vi "TestDownlink.vi"(1 "DL Tx  Power":dbl=-100.0, 2 "FPGA Reference":refnum<k20>, 3 "DL Data Rate":dbl=600.0 format="%.2f", 4 "DL Tx Freq":i64=905193250, 5 "error in":errorcluster {"code" format="%.0x"}, 6 "DL Rx Timeout (ms)":u32=60, 7 "Resp Timeout (ms)":i32 min=0, 9 "SMU Reference in":refnum<k15>, 10 "DL Rx Freq (Hz)":i64=905200000, 11 "Active Dut":T1, 12 "DL Freq Offset (Hz)":i64=6750, 13 "DxSupply":string="0") -> (14 "Set DL OK":bool, 15 "DL RSSI (dBm)":i16, 16 "Received Text":string, 17 "Get DL OK":bool, 18 "Meas DL Idd":dbl format="%0.5f", 19 "error out":errorcluster)   [LabVIEW 2018]
uses:
  Resources_Test/UART/ControlTestSlot.ctl
  <instrlib>/niRFSG/niRFSG.llb/niRFSG Ref Clock Sources.ctl
panel:
  out "Loop Index":i32
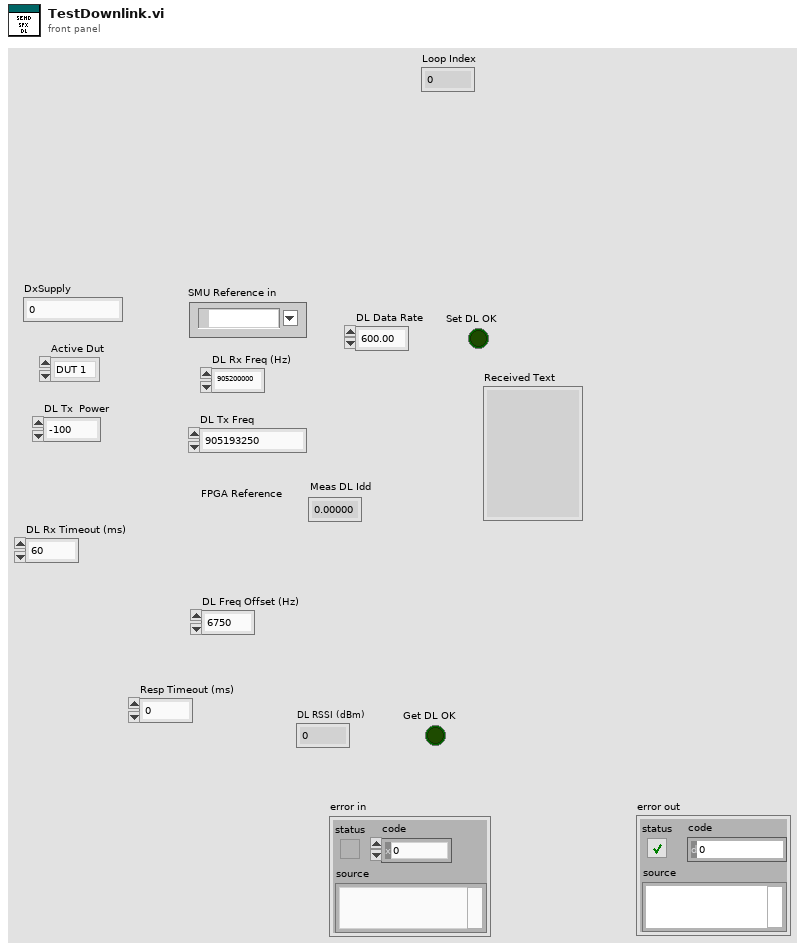
[diagram p1: front panel]
types:
  T1 = typedef "ControlTestSlot.ctl" = enum16{"DUT 1", "DUT 2"}
  T2 = typedef "niRFSG Ref Clock Sources.ctl" = string
  T3 = typedef "niAMT.lvlib/Complex Data Waveform.ctl" = cluster{"t0":dbl, "dt":dbl, "Y":cdb[]}
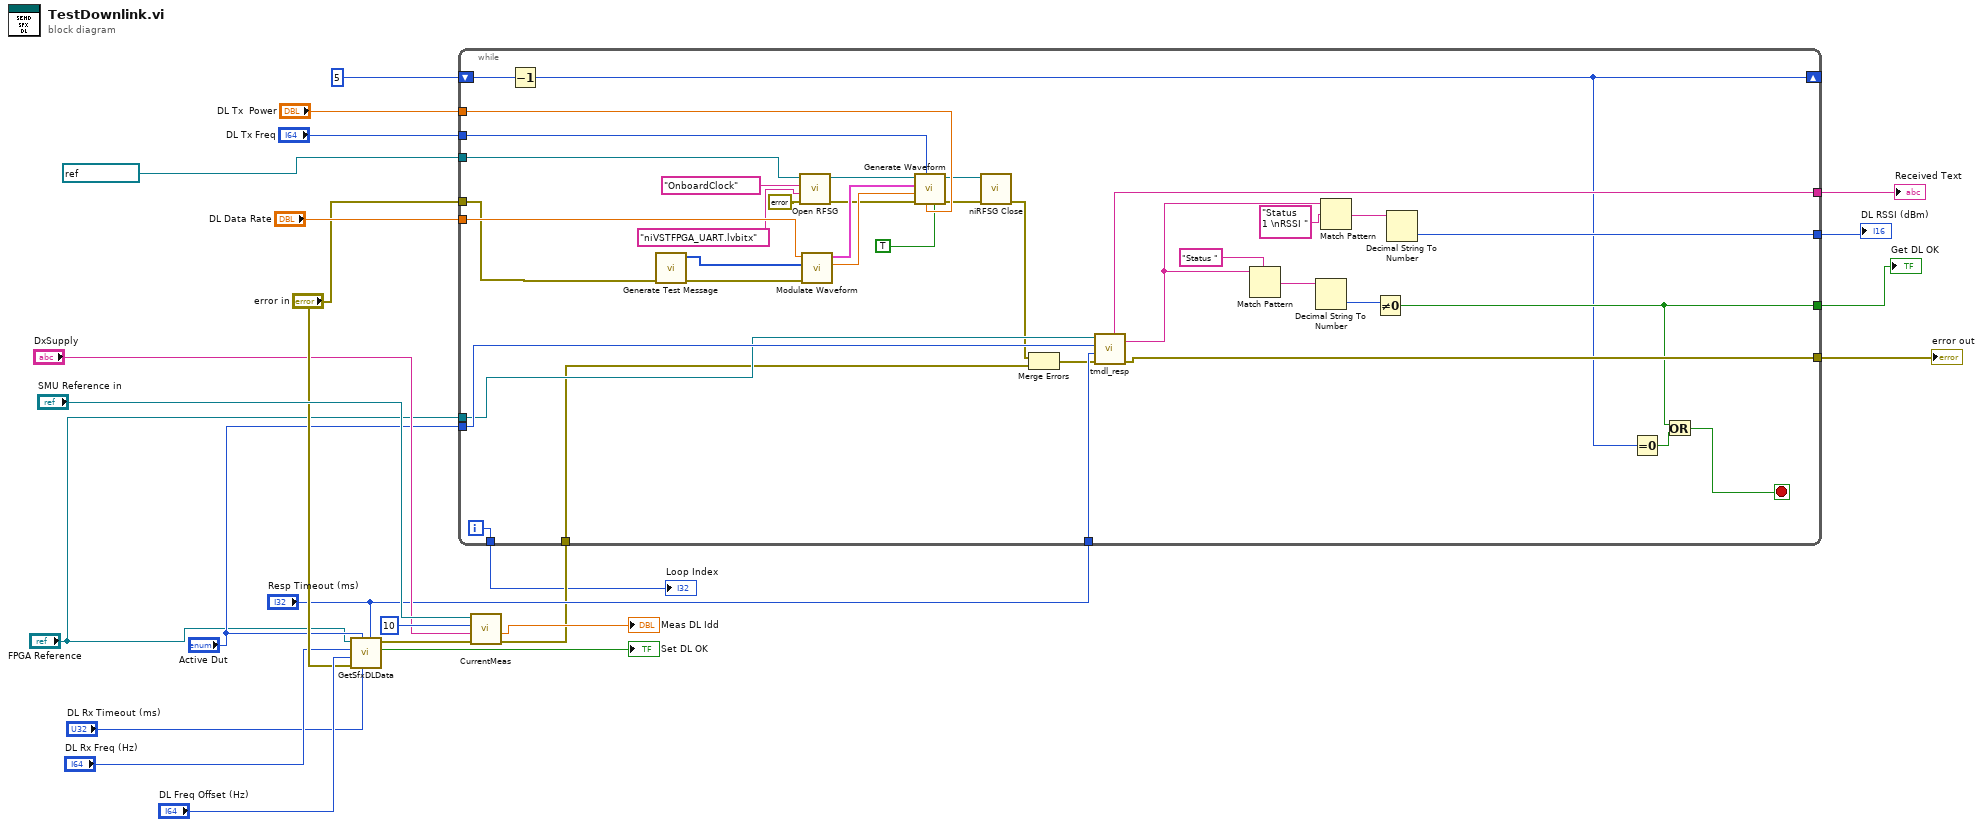
[diagram p0: block diagram]
diagram:
  n1 = call "GetSfxDLData.vi"("Resp Timeout (ms)"="Resp Timeout (ms)", "Rx Timeout (ms)"="DL Rx Timeout (ms)", "Enum"="Active Dut", "Error In"="error in", "Freq Offset (Hz)"="DL Freq Offset (Hz)", "Rx Freq (Hz)"="DL Rx Freq (Hz)", "FPGA Reference"="FPGA Reference") -> ("Error Out"=w20:errorcluster, "Get DL OK"=→"Set DL OK":bool)  [unwired: 3 out]
  n2 = call "CurrentMeas.vi"("error in (no error)"=w20, "DxSupply"="DxSupply", "Measure Record Length"=10, "instrument handle"="SMU Reference in") -> ("error out"=w7:errorcluster, "Idd Peak"=→"Meas DL Idd":dbl)  [unwired: 4 in, 2 out]
  n3 = while {
    tunnel: "DL Tx  Power" -> [w61]
    tunnel: "DL Data Rate" -> [w60]
    tunnel: "DL Tx Freq" -> [w59]
    tunnel: refnum<k15> "PXI1Slot5" ("RFSG Reference in") -> [w58]
    tunnel: "error in" -> [w57]
    tunnel: "Resp Timeout (ms)" -> [w55]
    tunnel: "Active Dut" -> [w54]
    tunnel: "FPGA Reference" -> [w53]
    tunnel: w7 -> [w52]
    tunnel: [w30] -> w5
    tunnel: [w29] -> w4
    tunnel: [w28] -> w3
    tunnel: [w27] -> w2
    shift-right: [w26] -> _
    shift-left: 5 -> [w32]
    tunnel: [w25] -> w1
    i -> [w25]
    stop <- w56 stop-if-true
    n4 = Decrement(x=w32) -> (x-1=w26:i32)
    n5 = call "Generate Test Message.vi"("error in"=w57) -> ("error out"=w41:errorcluster, "Output Bit Stream"=w40:i8[])  [unwired: 9 in]
    n6 = call "Open RFSG.vi"("error in"=errorcluster {"status"=FALSE, "code"=0, "source"=""}, "Bitfile"="niVSTFPGA_UART.lvbitx" ("Option String"), "Clock Source"=T2 "OnboardClock", "Resource Name"=w58) -> ("error out"=w47:errorcluster, "IVI Refnum out"=w46:refnum<k15>)  [unwired: 6 in]
    n7 = call "Modulate Waveform.vi"("error in"=w41, "input bit stream"=w40, "Symbol Rate, Hz"=w60) -> ("Signal Bandwidth"=w51:dbl, "output complex waveform"=w50:T3)  [unwired: 5 in, 2 out]
    n8 = call "Generate Waveform.vi"("Boolean"=TRUE, "Power Level (dBm)"=w61, "Center Frequency (Hz)"=w59, "error in (no error)"=w47, "Signal Bandwidth (Hz)"=w51, "IQ waveform"=w50, "IVI Refnum in"=w46) -> ("error out"=w44:errorcluster, "IVI Refnum out"=w45:refnum<k15>)  [unwired: 3 in]
    n9 = call <instrlib>:"niRFSG Close.vi"("instrument handle"=w45, "error in"=w44) -> ("error out"=w33:errorcluster)  [unwired: 13 in]
    n10 = Merge Errors(w33, w52) -> (w39:errorcluster)
    n11 = call "tmdl_resp.vi"("error in (no error)"=w39, "DL Rx Timeout (ms)"=w55, "Active Dut"=w54, "Refnum in"=w53) -> ("error out"=w30:errorcluster, "Received Text"=w29:string)  [unwired: 5 in, 1 out]
    n12 = Match Pattern(string=w29, regular expression="Status ") -> (after substring=w37:string)  [unwired: 1 in, 3 out]
    n13 = Decimal String To Number(string=w37) -> (number=w36:i32)  [unwired: 2 in, 1 out]
    n14 = Match Pattern(string=w29, regular expression="Status 1 \nRSSI ") -> (after substring=w38:string)  [unwired: 1 in, 3 out]
    n15 = Not Equal To 0?(x=w36) -> (x != 0?=w27:bool)
    n16 = Decimal String To Number(string=w38) -> (number=w28:i32)  [unwired: 2 in, 1 out]
    n17 = Equal To 0?(x=w26) -> (x = 0?=w31:bool)
    n18 = Or(x=w27, y=w31) -> (x .or. y?=w56:bool)
  }
  "error out" <- w5
  "Get DL OK" <- w2
  "DL RSSI (dBm)" <- w3
  "Received Text" <- w4
  "Loop Index" <- w1
